vi "TestGetScaleDataVI.vi"() -> ()   [LabVIEW 2017]
panel:
  out "error out":errorcluster
  out "Image Out":T1(plugin-control)
  in  "Original Image":path
  in  "Grid Descriptor":cluster{"X Step":sgl, "Y Step":sgl, "Unit":T2}={"X Step"=5.0, "Y Step"=5.0, "Unit"=enum."Millimeter"}
  in  "Calibration Image":path
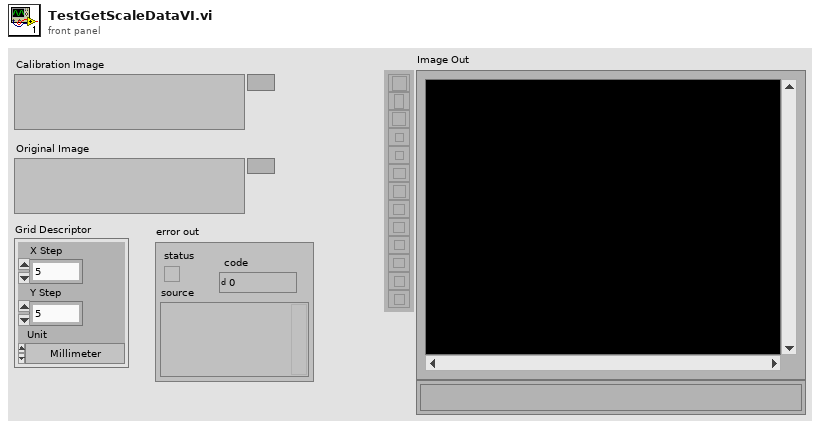
[diagram p1: front panel]
types:
  T1 = typedef "IMAQ Image.ctl" = refnum<image>
  T2 = typedef "Image Unit" = enum32{"Undefined", "Angström", "Micrometer", "Millimeter", "Centimeter", "Meter", "Kilometer", "Microinch", "Inch", "Feet", "Nautical miles", "Standard miles", "Steps"}
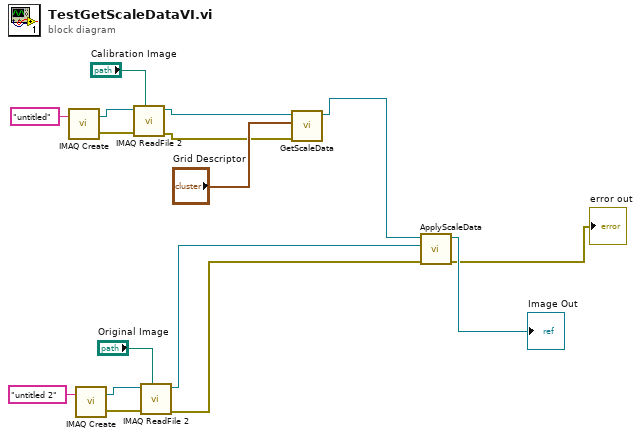
[diagram p0: block diagram]
diagram:
  n1 = call "IMAQ Create"("Image Name"="untitled") -> ("New Image"=w14:T1, "error out"=w13:errorcluster)  [unwired: 4 in]
  n2 = call "IMAQ Create"("Image Name"="untitled 2") -> ("New Image"=w7:T1, "error out"=w6:errorcluster)  [unwired: 4 in]
  n3 = call "IMAQ ReadFile 2"("File Path"="Calibration Image", "error in (no error)"=w13, "Image"=w14) -> ("error out"=w11:errorcluster, "Image Out"=w10:T1)  [unwired: 4 in, 3 out]
  n4 = call "IMAQ ReadFile 2"("File Path"="Original Image", "error in (no error)"=w6, "Image"=w7) -> ("error out"=w1:errorcluster, "Image Out"=w5:T1)  [unwired: 4 in, 3 out]
  n5 = call "GetScaleData.vi"("error in (no error)"=w11, "Grid Descriptor"="Grid Descriptor", "Image Src"=w10) -> ("Image"=w4:T1)  [unwired: 7 in, 1 out]
  n6 = call "ApplyScaleData.vi"("error in (no error)"=w1, "Image Dst"=w5, "Image Src"=w4) -> ("error out"=→"error out":errorcluster, "Corrected Image"=→"Image Out":T1)  [unwired: 7 in]
